vi "MaskFromARGB.vi"(8 "error in (no error)":errorcluster, 9 "Value":T1={"Alpha"=255, "RGB"=0}, 10 "Mask Destination":refnum<data-value>, 11 "ARGB Image Source":refnum<data-value>) -> (0 "error out":errorcluster, 3 "Mask Destination (duplicate)":refnum<data-value>)   [LabVIEW 2020, in "g_ar_toolkit.image.lvlib"]
uses:
  g_ar_toolkit.image.lvlib
  ARGB Colour.ctl
  <vilib>/Utility/error.llb/Error Cluster From Error Code.vi
  5701baee-35e2-4306-9a77-a9fdbb5b3a7f.vi
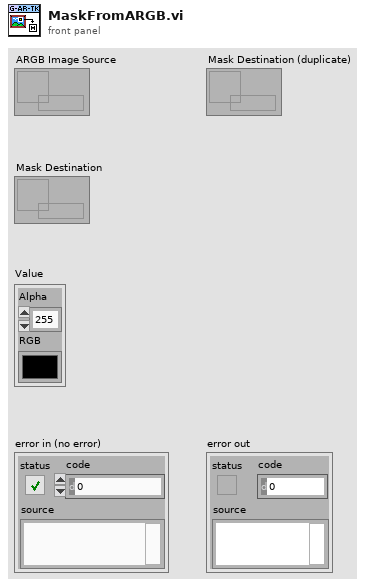
[diagram p1: front panel]
types:
  T1 = typedef "g_ar_toolkit.image.lvlib/ARGB Colour.ctl" = cluster{"Alpha":u8, "RGB":u32}
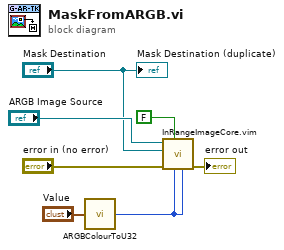
[diagram p0: block diagram]
diagram:
  n1 = call "ARGBColourToU32.vi"("ARGB Colour"="Value") -> ("U32 Colour"=w1:u32)
  n2 = call "InRangeImageCore.vim"("Upper"=w1, "Lower"=w1, "IgnoreAlpha"=FALSE, "error in (no error)"="error in (no error)", "In-Range-Result"="Mask Destination", "Src"="ARGB Image Source") -> ("error out"=→"error out":errorcluster)  [unwired: 5 in]
  "Mask Destination (duplicate)" <- "Mask Destination"
